vi "Init Health.vi"(8 "error in (no error)":errorcluster, 11 "System Health Module in":refnum<class "System Health Module.lvclass">) -> (0 "error out":errorcluster, 3 "System Health Module out":refnum<class "System Health Module.lvclass">)   [LabVIEW 2020, in "Volatus.lvlib" / "System Health Module.lvclass"]
uses:
  System Health Module.lvclass
  C:/dev/lv20CE/relink/lv-volatus/Volatus/Module/Module.lvclass
  Event Level.ctl
  Module/Module.lvclass/Module.ctl
  Module/Module.lvclass
  System Health Module.lvclass/System Health Module.ctl
  Volatus.lvlib
  C:/dev/lv20CE/relink/lv-volatus/Volatus/System Health Module/System Health Module.lvclass
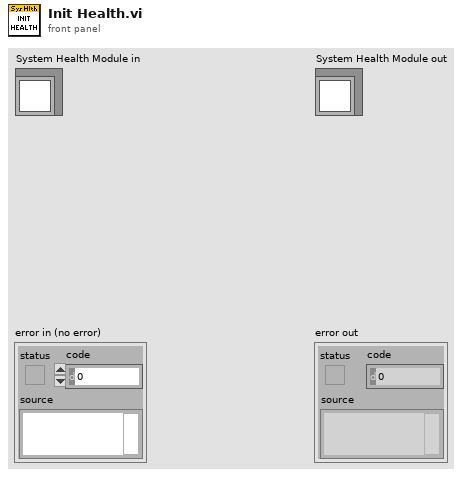
[diagram p1: front panel]
types:
  T1 = typedef "Volatus.lvlib/Event Level.ctl" = enum16{"Debug", "Info", "Warning", "Error"}
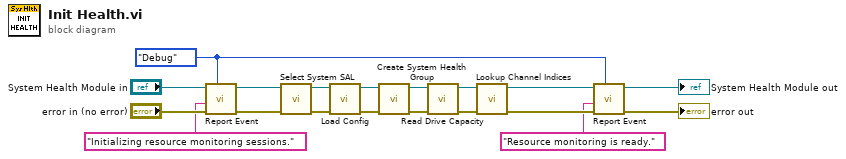
[diagram p0: block diagram]
diagram:
  w8 = Event_Level."Debug" ("Level (Info)")
  n1 = call "Report Event.vi"("Level (Info)"=w8, "error in (no error)"="error in (no error)", "Message"="Initializing resource monitoring sessions.", "Module in"="System Health Module in") -> ("error out"=w15:errorcluster, "Module out"=w13:refnum<class "System Health Module.lvclass">)  [unwired: 6 in]
  n2 = call "Select System SAL.vi"("error in (no error)"=w15, "System Health Module in"=w13) -> ("error out"=w19:errorcluster, "System Health Module out"=w18:refnum<class "System Health Module.lvclass">)  [unwired: 8 in]
  n3 = call "Load Config.vi"("error in (no error)"=w19, "System Health Module in"=w18) -> ("error out"=w5:errorcluster, "System Health Module out"=w6:refnum<class "System Health Module.lvclass">)  [unwired: 8 in]
  n4 = call "Create System Health Group.vi"("error in (no error)"=w5, "System Health Module in"=w6) -> ("error out"=w4:errorcluster, "System Health Module out"=w3:refnum<class "System Health Module.lvclass">)  [unwired: 8 in]
  n5 = call "Read Drive Capacity.vi"("error in (no error)"=w4, "System Health Module in"=w3) -> ("error out"=w2:errorcluster, "System Health Module out"=w1:refnum<class "System Health Module.lvclass">)  [unwired: 8 in]
  n6 = call "Lookup Channel Indices.vi"("error in (no error)"=w2, "System Health Module in"=w1) -> ("error out"=w16:errorcluster, "System Health Module out"=w10:refnum<class "System Health Module.lvclass">)  [unwired: 8 in]
  n7 = call "Report Event.vi"("Level (Info)"=w8, "error in (no error)"=w16, "Message"="Resource monitoring is ready.", "Module in"=w10) -> ("error out"=→"error out":errorcluster, "Module out"=→"System Health Module out":refnum<class "System Health Module.lvclass">)  [unwired: 6 in]
